vi "construct.vi"(8 "error in (no error)":errorcluster, 9 "configuration name":string, 10 "load config file?":bool=TRUE, 11 "GenericPlugin in":refnum<class "GenericComponent.lvclass">) -> (0 "error out":errorcluster, 3 "GenericPlugin out":refnum<class "GenericComponent.lvclass">)   [LabVIEW 2010, in "GenericComponent.lvclass"]
uses:
  GenericComponent.lvclass
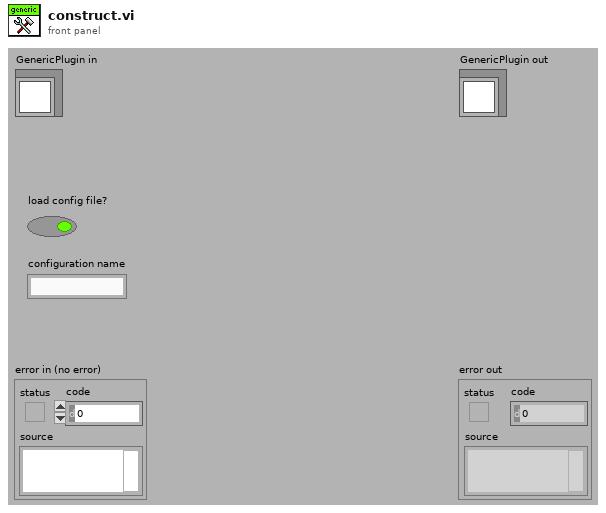
[diagram p1: front panel]
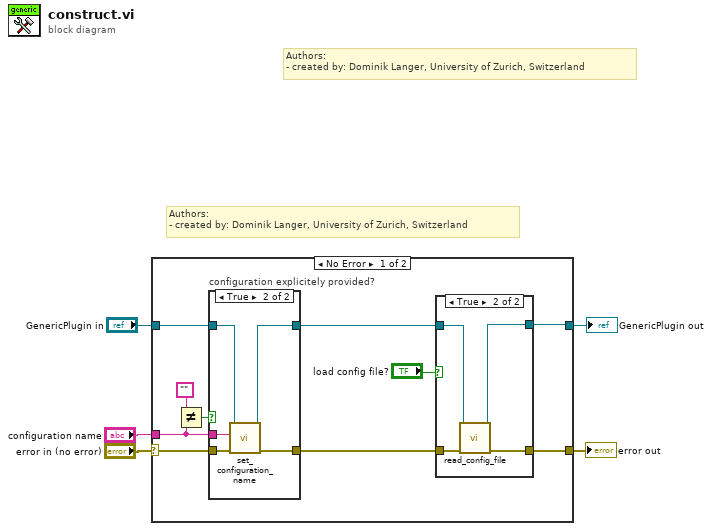
[diagram p0: block diagram]
diagram:
  # "Authors: \n- created by: Dominik Langer, University of Zurich, Switzerland"
  # "Authors: \n- created by: Dominik Langer, University of Zurich, Switzerland"
  n1 = case shown="No Error" "error in (no error)" {
    selector: "error in (no error)" -> [w15 w30]
    tunnel: [w10 w30] -> w4
    tunnel: [w11 w29] -> w2
    tunnel: "GenericPlugin in" -> [w13 w29]
    tunnel: "configuration name" -> [w9 _]
    frame No Error {
      n2 = Not Equal?(x="", y=w9) -> (x != y?=w7:bool)
      n3 = case "configuration explicitely provided?" shown="True" w7 {
        tunnel: w15 -> [w16 w22]
        tunnel: [w16 w21] -> w14
        tunnel: w13 -> [w17 w20]
        tunnel: [w17 w19] -> w6
        tunnel: w9 -> [_ w18]
        frame False {
        }
        frame True {
          n4 = call-dynamic "set_configuration_name.vi"("error in (no error)"=w22, "configuration"=w18, "GenericPlugin.lvclass in"=w20) -> ("error out"=w21:errorcluster, "GenericPlugin.lvclass out"=w19:refnum<class "GenericComponent.lvclass">)  [unwired: 7 out]
        }
      }
      n5 = case shown="True" "load config file?" {
        tunnel: w14 -> [w23 w28]
        tunnel: [w23 w27] -> w10
        tunnel: w6 -> [w24 w26]
        tunnel: [w24 w25] -> w11
        frame False {
        }
        frame True {
          n6 = call-dynamic "read_config_file.vi"("error in (no error)"=w28, "GenericPlugin in"=w26) -> ("error out"=w27:errorcluster, "GenericPlugin out"=w25:refnum<class "GenericComponent.lvclass">)  [unwired: 1 in, 7 out]
        }
      }
    }
    frame Error {
    }
  }
  "error out" <- w4
  "GenericPlugin out" <- w2
